vi "Find VI Path.vi"(8 "error in (no error)":errorcluster, 10 "XML path (absolute)":path, 11 "VI Panel Layout in":refnum<class "VI Panel Layout.lvclass">) -> (0 "error out":errorcluster, 1 "keyword":string, 2 "VI path (absolute)":path, 3 "VI Panel Layout out":refnum<class "VI Panel Layout.lvclass">)   [LabVIEW 2010, in "NI_SE_Front Panel Layout.lvlib" / "VI Panel Layout.lvclass"]
uses:
  VI Panel Layout.lvclass
  VI Panel Layout.lvclass/VI Panel Layout.ctl
  File Name to Width_Height.vi
  <vilib>/Utility/libraryn.llb/Check if File or Folder Exists.vi
  NI_SE_Front Panel Layout.lvlib
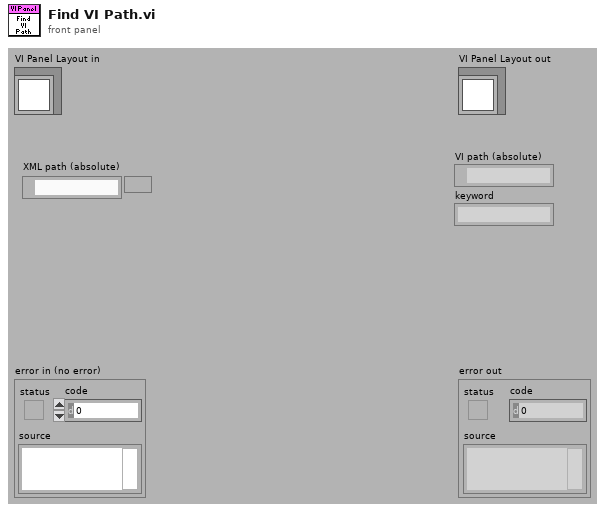
[diagram p1: front panel]
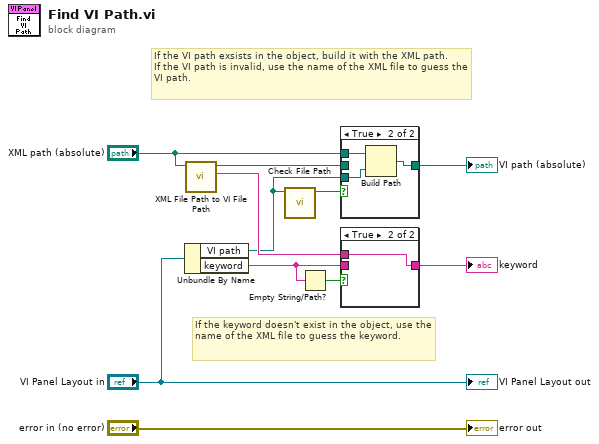
[diagram p0: block diagram]
diagram:
  # "If the keyword doesn't exist in the object, use the name of the XML file to guess the keyword."
  # "If the VI path exsists in the object, build it with the XML path.\nIf the VI path is invalid, use the name of the XML file to guess the VI path."
  n1 = Unbundle By Name("VI Panel Layout in") -> ("VI path"=w1:path, "keyword"=w3:string)
  n2 = call "XML File Path to VI File Path.vi"("XML file path"="XML path (absolute)") -> ("keyword"=w2:string, "VI file path"=w5:path)  [unwired: 9 in]
  n3 = call "Check File Path.vi"("path"=w1) -> ("valid path?"=w6:bool)  [unwired: 9 in, 1 out]
  n4 = Empty String/Path?(string/path=w3) -> (empty?=w4:bool)
  n5 = case shown="True" w6 {
    tunnel: w1 -> [_ w14]
    tunnel: "XML path (absolute)" -> [_ w15]
    tunnel: [w12 w13] -> w8
    tunnel: w5 -> [w12 _]
    frame False {
    }
    frame True {
      n6 = Build Path(base path=w15, name or relative path=w14) -> (appended path=w13:path)
    }
  }
  "VI path (absolute)" <- w8
  n7 = case shown="True" w4 {
    tunnel: w3 -> [w16 _]
    tunnel: w2 -> [_ w17]
    tunnel: [w16 w17] -> w7
    frame False {
    }
    frame True {
    }
  }
  "keyword" <- w7
  "error out" <- "error in (no error)"
  "VI Panel Layout out" <- "VI Panel Layout in"
